vi "SPD.Config Read Test04 DCR.vi"(8 "Error In":errorcluster, 11 "SPD.Stand Ctrl in":T2 {"spdDeviceSession"."hidSPD.Sturtup Values"."HV_bias" format="%#_6p, V"; "spdDeviceSession"."hidSPD.Sturtup Values"."TSet" format="%#_6p, DegC"; "spdDeviceSession"."hidSPD.Controller"."HV_bias" format="%#_6p, V"; "spdDeviceSession"."hidSPD.Controller"."TSet" format="%#_6p, DegC"}) -> (0 "Error Out":errorcluster, 2 "DCR Meas Params":T1, 3 "SPD.Stand Ctrl out":T2 {"spdDeviceSession"."hidSPD.Sturtup Values"."HV_bias" format="%#_6p, V"; "spdDeviceSession"."hidSPD.Sturtup Values"."TSet" format="%#_6p, DegC"; "spdDeviceSession"."hidSPD.Controller"."HV_bias" format="%#_6p, V"; "spdDeviceSession"."hidSPD.Controller"."TSet" format="%#_6p, DegC"})   [LabVIEW 2018]
uses:
  typedefs/SPD.Stand Ctrl.ctl
  Instruments/SPD HID Interface/hidSPDLibForLabView/LibVIs/hidSPD Controls/hidSPD Device Session.ctl
  Instruments/SPD HID Interface/hidSPDLibForLabView/LibVIs/hidSPD Controls/hidSPD Controller.ctl
  Instruments/SPD HID Interface/hidSPDLibForLabView/LibVIs/hidSPD Controls/hidSPD SPD Type.ctl
  Instruments/KC705 DevBoard/typedefs/DevB.Session.ctl
  Instruments/KeySight 53230A/typedefs/FreqC.Session.ctl
  Instruments/KeySight 8164B/KeySight 8164B LAN InstrLib/typedefs/KeySight 8164B control.ctl
  Instruments/LeCroy SDA830/typedefs/LeCroy.Session.ctl
  typedefs/SPD.Events.ctl
  SPD.Config File ctrl.ctl
  <vilib>/Utility/config.llb/Config Data RefNum.ctl
  typedefs/SPD.Meas Result.ctl
  typedefs/SPD.Queues.ctl
  typedefs/SPD.Stand state.ctl
  SPD Measurements/DCR/typedefs/SPD.DCR Test Params.ctl
  <vilib>/Utility/config.llb/Read Key (I32).vi
  <vilib>/Utility/config.llb/Read Key (Double).vi
  <vilib>/Utility/config.llb/NI_LVConfig.lvlib
  Instruments/KeySight 8164B/KeySight 8164B LAN InstrLib.lvlib
  Instruments/SPD HID Interface/hidSPDLibForLabView/hidSPDLibForLabView.lvlib
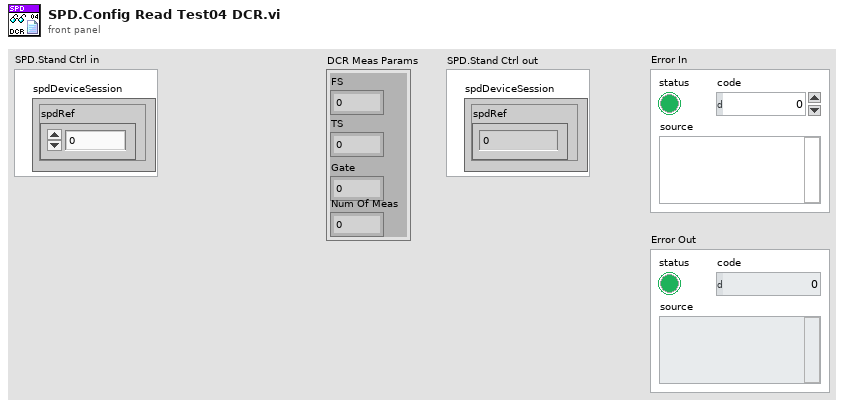
[diagram p1: front panel]
types:
  T1 = typedef "SPD.DCR Test Params.ctl" = cluster{"FS":i32, "TS":i32, "Gate":dbl, "Num Of Meas":i32}
  T2 = typedef "SPD.Stand Ctrl.ctl" = cluster{"spdDeviceSession":T3, "DevBSession":T6, "FreqCSession":T7, "8164BSession":T8, "LeCroySession":T9, "Events":T10, "configFile":T11, "SPD.Result":T13, "SPD.Queues":T14, "Console":refnum<vi>}
  T3 = typedef "hidSPDLibForLabView.lvlib/hidSPD Device Session.ctl" = cluster{"spdRef":u64, "connected":bool, "spdName":string, "hidSPD.Controller":T4, "hidSPD.Sturtup Values":T4, "SPD Type":T5}
  T4 = typedef "hidSPDLibForLabView.lvlib/hidSPD Controller.ctl" = cluster{"TSet":sgl, "HV_bias":sgl, "DDS_stb_code":u16}
  T5 = typedef "hidSPDLibForLabView.lvlib/hidSPD SPD Type.ctl" = enum16{"Free Run", "Strobe"}
  T6 = typedef "DevB.Session.ctl" = cluster{"DevBRef":refnum<visa-resource-name>, "connected":bool}
  T7 = typedef "FreqC.Session.ctl" = cluster{"FreqCRef":refnum<visa-resource-name>, "timeout":dbl, "Gate":dbl, "connected":bool}
  T8 = typedef "KeySight 8164B LAN InstrLib.lvlib/KeySight 8164B control.ctl" = cluster{"Connection ID":refnum<k5>, "Connected":bool, "Info":string, "Slots Info":string[]}
  T9 = typedef "LeCroy.Session.ctl" = cluster{"LeCroySession":refnum<visa-resource-name>, "connected":bool}
  T10 = typedef "SPD.Events.ctl" = cluster{"DCRTest":refnum<user-event>, "Stop":refnum<user-event>}
  T11 = typedef "SPD.Config File ctrl.ctl" = cluster{"configFile ref":T12, "configFile path":path, "equipmentFile ref":T12}
  T12 = typedef "NI_LVConfig.lvlib/Config Data RefNum.ctl" = refnum<k1>
  T13 = typedef "SPD.Meas Result.ctl" = cluster{"HV_Bias":dbl[][][], "Stb_code":dbl[], "Temprature":dbl[], "Data":dbl[][][][], "DateTime":string}
  T14 = typedef "SPD.Queues.ctl" = cluster{"state queue":refnum<queue>}
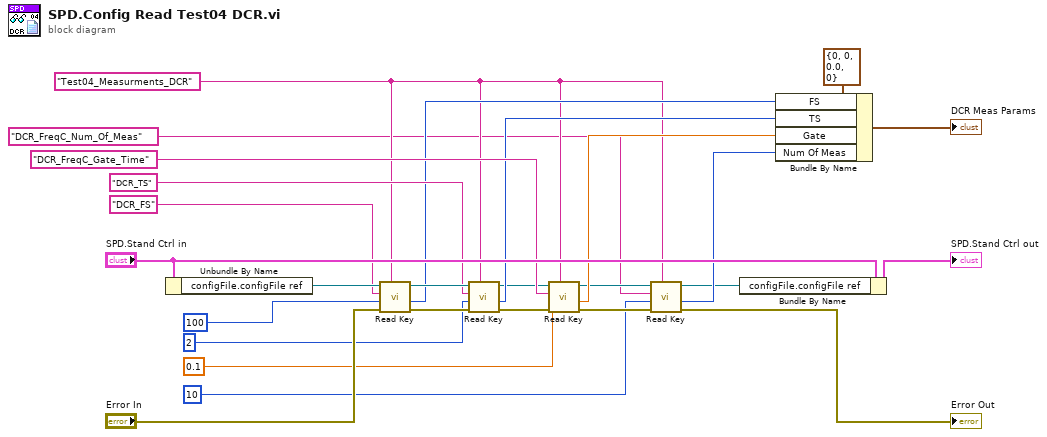
[diagram p0: block diagram]
diagram:
  w10 = "Test04_Measurments_DCR" ("section")
  n1 = Unbundle By Name("SPD.Stand Ctrl in") -> ("configFile.configFile ref"=w25:T12)
  n2 = call-poly <vilib>:"Read Key.vi"("section"=w10, "error in (no error)"="Error In", "default value"=100, "key"="DCR_FS", "refnum"=w25) -> ("error out"=w21:errorcluster, "value"=w15:i32, "refnum out"=w20:T12)  [unwired: 3 in, 1 out]
  n3 = call-poly <vilib>:"Read Key.vi"("section"=w10, "error in (no error)"=w21, "default value"=2, "key"="DCR_TS", "refnum"=w20) -> ("error out"=w4:errorcluster, "value"=w14:i32, "refnum out"=w5:T12)  [unwired: 3 in, 1 out]
  n4 = call-poly <vilib>:"Read Key.vi"("section"=w10, "error in (no error)"=w4, "default value"=0.1, "key"="DCR_FreqC_Gate_Time", "refnum"=w5) -> ("error out"=w9:errorcluster, "value"=w13:dbl, "refnum out"=w11:T12)  [unwired: 3 in, 1 out]
  n5 = call-poly <vilib>:"Read Key.vi"("section"=w10, "error in (no error)"=w9, "default value"=10, "key"="DCR_FreqC_Num_Of_Meas", "refnum"=w11) -> ("error out"=→"Error Out":errorcluster, "value"=w8:i32, "refnum out"=w3:T12)  [unwired: 3 in, 1 out]
  n6 = Bundle By Name(cluster="SPD.Stand Ctrl in", "configFile.configFile ref"=w3) -> (→"SPD.Stand Ctrl out":T2)
  n7 = Bundle By Name(cluster=T1 {"FS"=0, "TS"=0, "Gate"=0.0, "Num Of Meas"=0} ("DCRParams"), "FS"=w15, "TS"=w14, "Gate"=w13, "Num Of Meas"=w8) -> (→"DCR Meas Params":T1)
